vi "CRYGet Changed Ana Curve Name.vi"(0 "Old Name":string[](array[string]), 1 "Signal Tyep":string, 3 "Use Channel Name?":bool caption="Use Channel Name", 5 "Current Name":string[](array[string]), 7 "Changed Name Table in":string[][](array[string]), 9 "New Custom Type( Channel case)":string[](array[string]), 11 "Change State":bool, 12 "Load?":bool, 14 "Change Use Channel":bool) -> (10 "Changed Name Table  out":string[][](array[string]))   [LabVIEW 2013]
panel:
  out "Array":string[][](array[string])
  out "Changed Curve in":string[][](array[string])
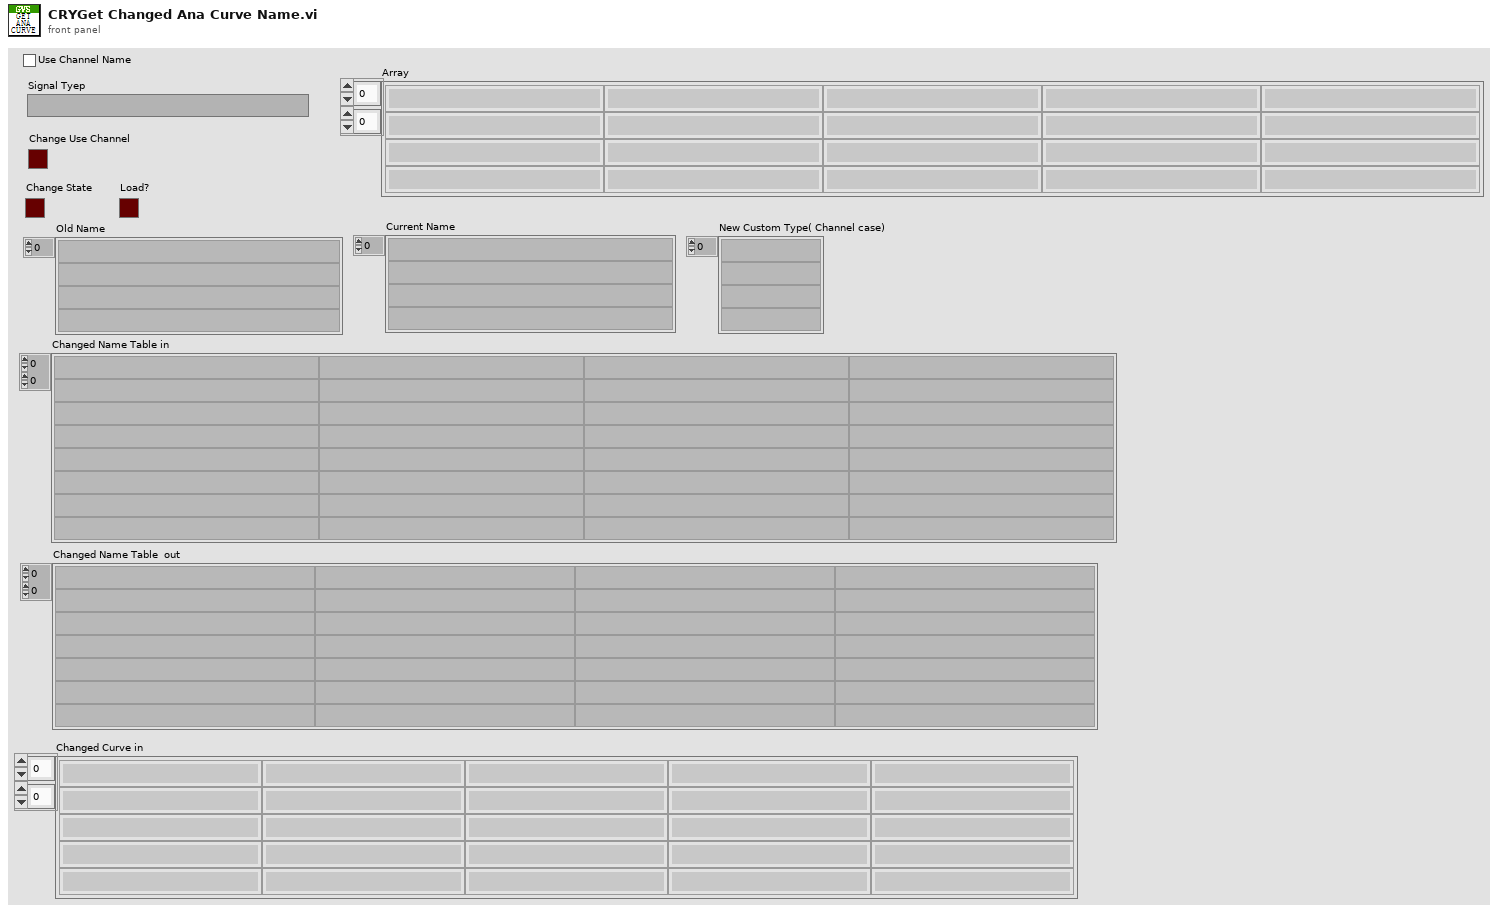
[diagram p1: front panel]
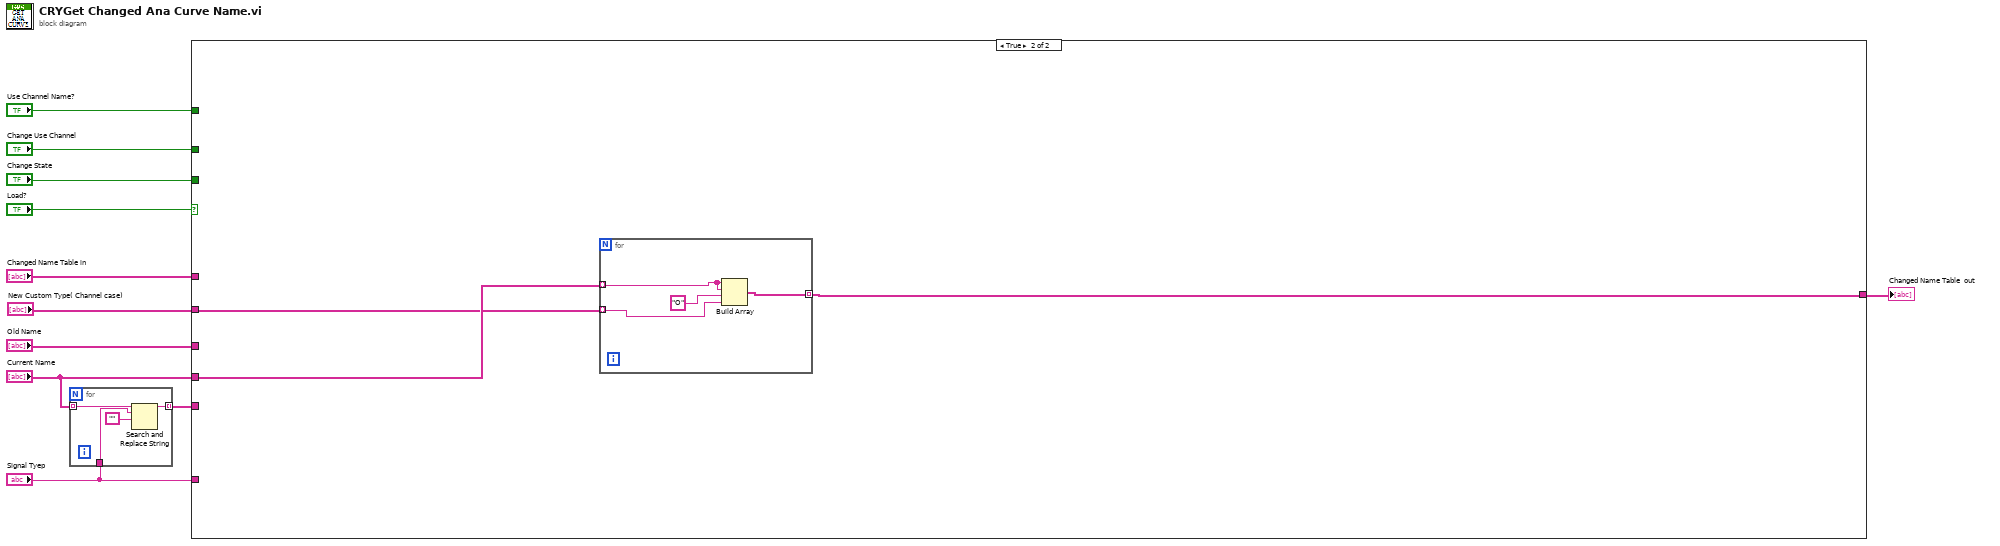
[diagram p0: block diagram]
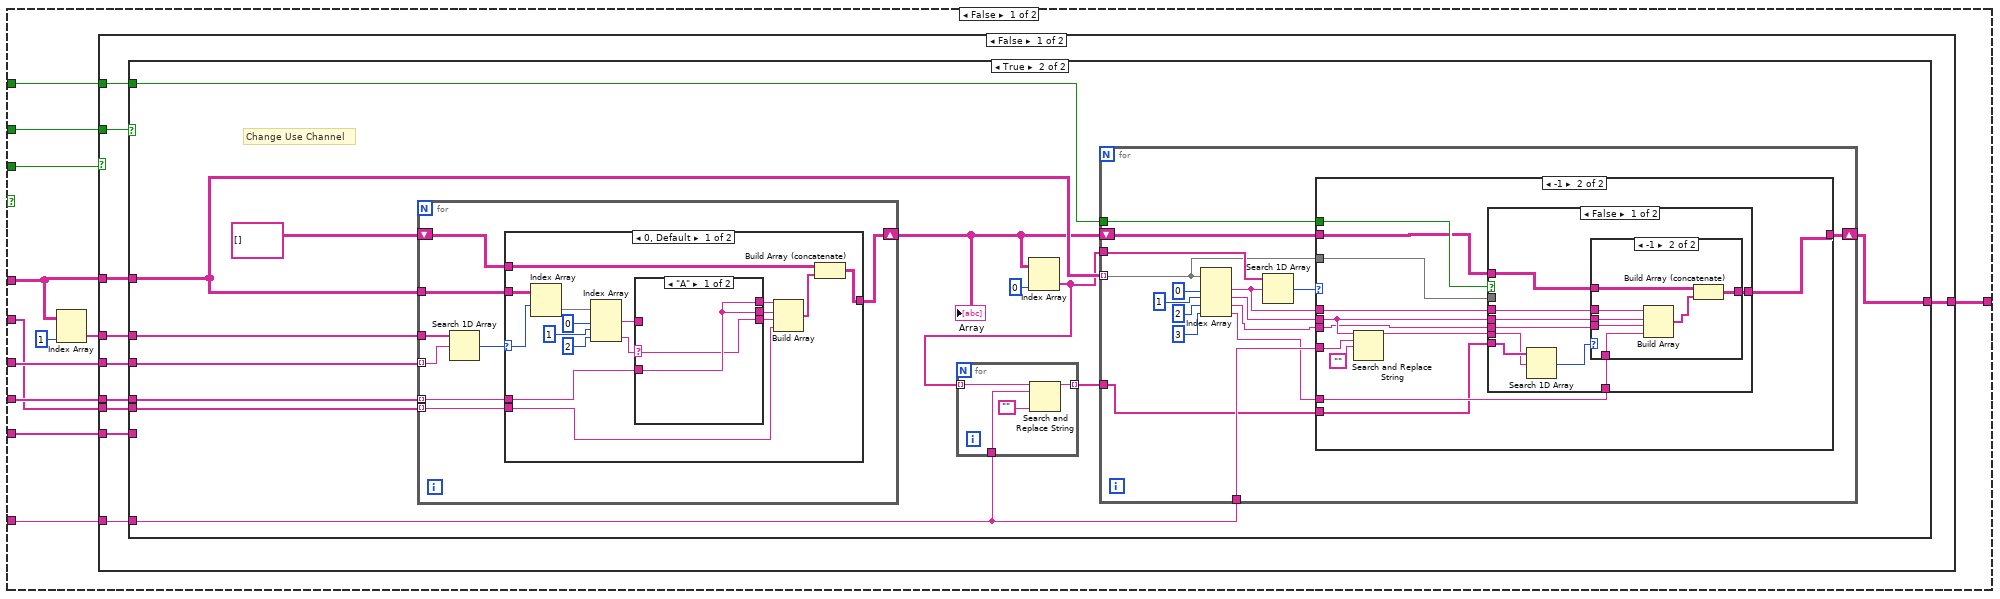
[diagram p2: hidden frame]
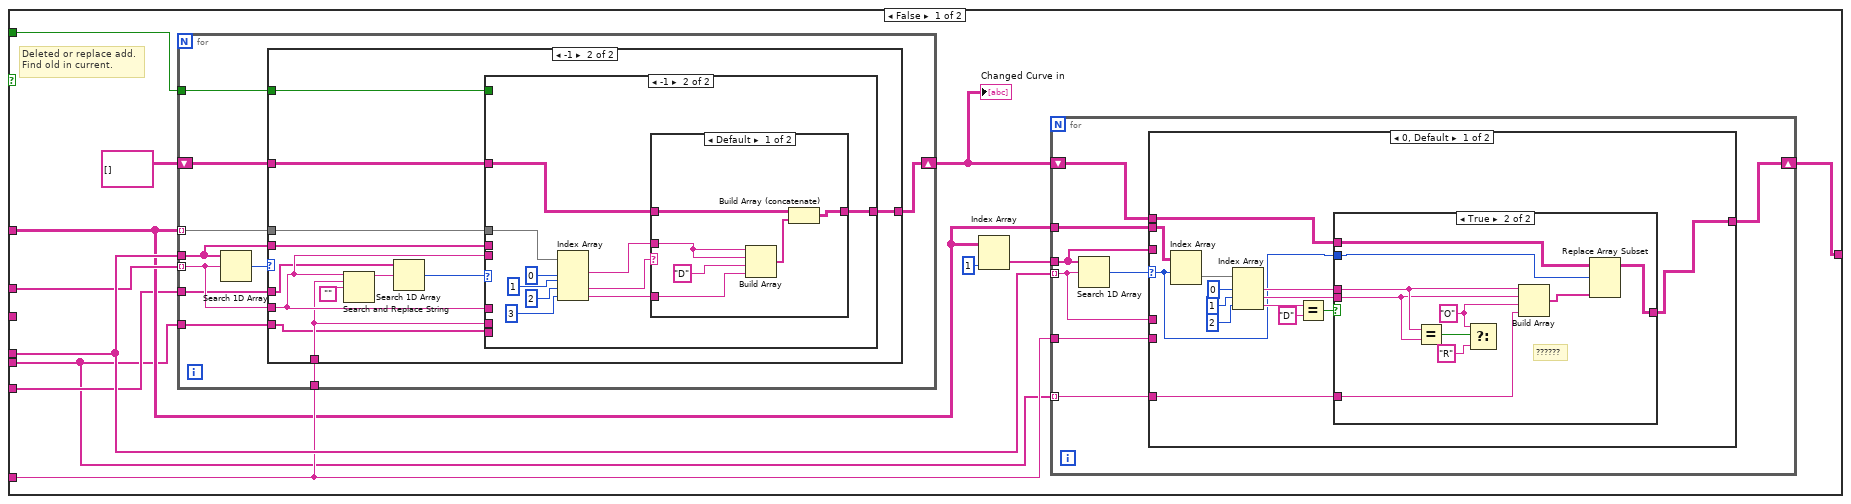
[diagram p3: hidden frame]
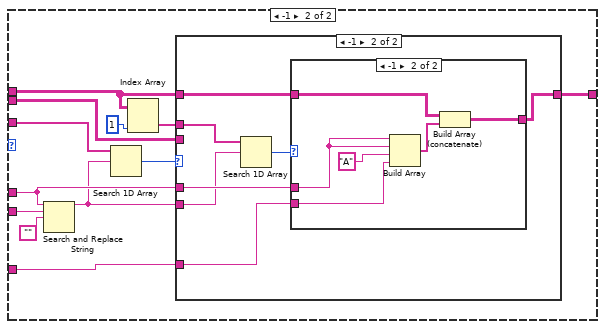
[diagram p5: hidden frame]
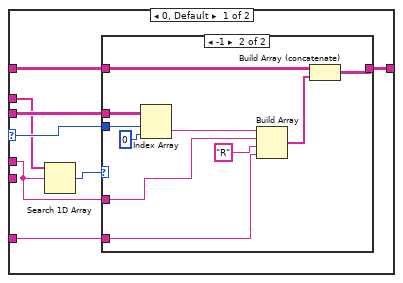
[diagram p6: hidden frame]
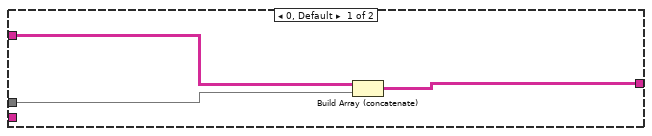
[diagram p9: hidden frame]
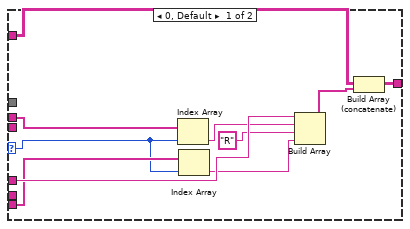
[diagram p10: hidden frame]
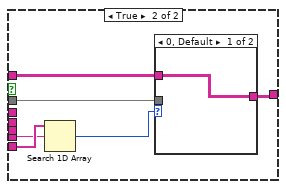
[diagram p14: hidden frame]
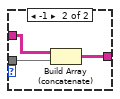
[diagram p15: hidden frame]
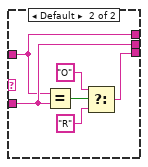
[diagram p16: hidden frame]
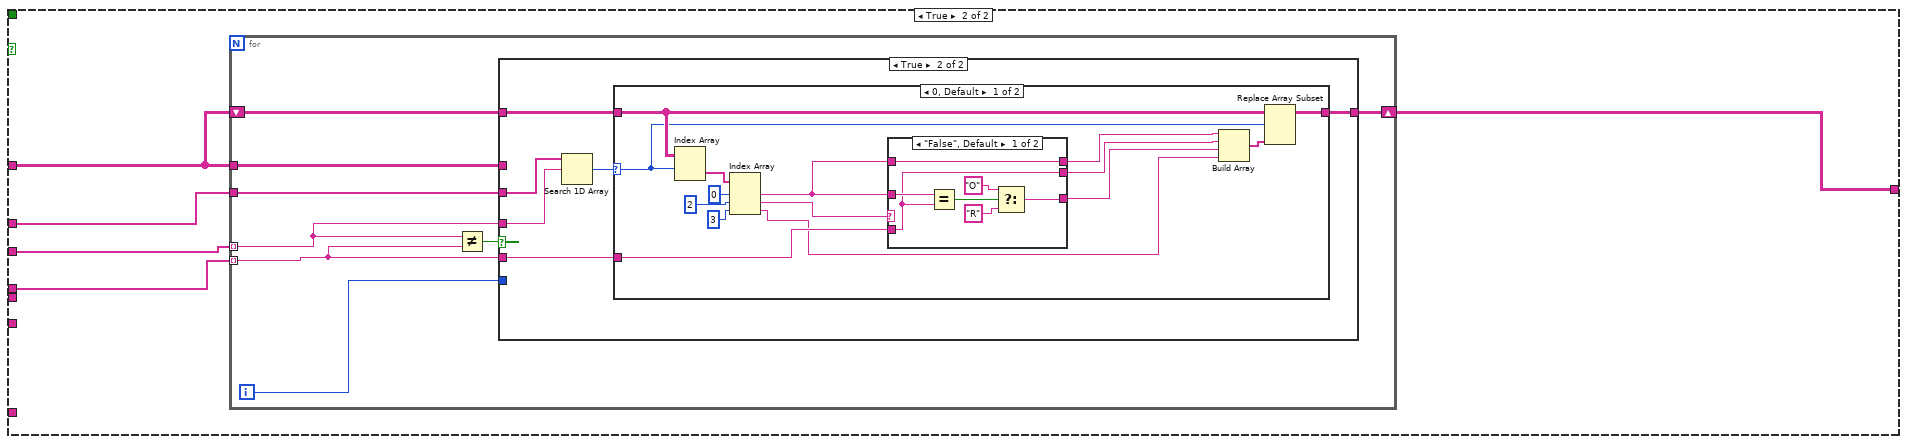
[diagram p18: hidden frame]
diagram:
  n1 = for {
    tunnel: "Current Name" -> [w14] mode=indexing
    tunnel: "Signal Tyep" -> [w13]
    tunnel: [w12] -> w2 mode=indexing
    n2 = Search and Replace String(input string=w14, search string=w13, replace string="" ("replace string (\"\")")) -> (result string=w12:string)  [unwired: 5 in, 3 out]
  }
  n3 = case shown="True" "Load?" {
    tunnel: [w27 w332] -> w11
    tunnel: "Changed Name Table in" -> [w25 _]
    tunnel: "Current Name" -> [w24 w333]
    tunnel: "Change State" -> [w23 _]
    tunnel: "Old Name" -> [w21 _]
    tunnel: "Change Use Channel" -> [w20 _]
    tunnel: "Signal Tyep" -> [w19 _]
    tunnel: "Use Channel Name?" -> [w18 _]
    tunnel: w2 -> [w17 _]
    tunnel: "New Custom Type( Channel case)" -> [w16 w331]
    frame False {
      n4 = Index Array(array=w25, index (col)=1 ("disabled index (col)")) -> (element=w22:string[])  [unwired: 1 in]
      n5 = case shown="False" w23 {
        tunnel: [w34 w286] -> w27
        tunnel: w22 -> [w36 w289]
        tunnel: w25 -> [w35 w287]
        tunnel: w24 -> [w37 w290]
        tunnel: w21 -> [w32 w288]
        tunnel: w20 -> [w33 _]
        tunnel: w19 -> [w31 _]
        tunnel: w18 -> [w30 _]
        tunnel: w17 -> [w29 _]
        tunnel: w16 -> [w28 _]
        frame False {
          n6 = case shown="True" w33 {
            tunnel: w37 -> [w48 w191]
            tunnel: w36 -> [w44 w189]
            tunnel: w35 -> [w40 w188]
            tunnel: [w47 w185] -> w34
            tunnel: w32 -> [_ w192]
            tunnel: w31 -> [w46 w182]
            tunnel: w30 -> [w45 w184]
            tunnel: w29 -> [w39 _]
            tunnel: w28 -> [w38 w183]
            frame False {
              # "Deleted or replace add.\nFind old in current."
              n7 = for {
                tunnel: w48 -> [w131]
                tunnel: w44 -> [w130] mode=indexing
                shift-right: [w136] -> w42
                shift-left: string[][] [] ("Changed Curve in") -> [w135]
                tunnel: w40 -> [w134] mode=indexing
                tunnel: w46 -> [w133]
                tunnel: w45 -> [w132]
                tunnel: w39 -> [w129]
                tunnel: w38 -> [w128]
                n8 = Search 1D Array(1D array=w131, element=w130) -> (index of element=w137:i32)  [unwired: 1 in]
                n9 = case shown="-1" w137 {
                  tunnel: [w139 w151] -> w136
                  tunnel: w135 -> [w140 w152]
                  tunnel: w134 -> [w138 w147]
                  tunnel: w133 -> [_ w143]
                  tunnel: w130 -> [_ w144]
                  tunnel: w132 -> [_ w145]
                  tunnel: w131 -> [_ w146]
                  tunnel: w129 -> [_ w142]
                  tunnel: w128 -> [_ w141]
                  frame 0, Default {
                    n10 = Build Array (concatenate)(w140, w138) -> (w139:string[][])
                  }
                  frame -1 {
                    n11 = Search and Replace String(input string=w144, search string=w143, replace string="" ("replace string (\"\")")) -> (result string=w149:string)  [unwired: 5 in, 3 out]
                    n12 = Search 1D Array(1D array=w142, element=w149) -> (index of element=w148:i32)  [unwired: 1 in]
                    n13 = case shown="-1" w148 {
                      selector: w148 -> [w154 _]
                      tunnel: w152 -> [w162 w172]
                      tunnel: [w161 w171] -> w151
                      tunnel: w147 -> [_ w167]
                      tunnel: w144 -> [w160 _]
                      tunnel: w145 -> [_ _]
                      tunnel: w143 -> [_ _]
                      tunnel: w146 -> [w159 _]
                      tunnel: w144 -> [_ _]
                      tunnel: w141 -> [w155 _]
                      frame 0, Default {
                        n14 = Index Array(array=w159, index=w154) -> (element=w156:string)
                        n15 = Index Array(array=w155, index=w154) -> (element=w153:string)
                        n16 = Build Array(w160, w156, "R" ("element"), w153) -> (w158:string[])
                        n17 = Build Array (concatenate)(w162, w158) -> (w161:string[][])
                      }
                      frame -1 {
                        n18 = Index Array(array=w167, index #1=0 ("index"), index #2=1 ("index"), index #3=2 ("index"), index #4=3 ("index")) -> (element #1=w166:string, element #3=w165:string, element #4=w163:string)  [unwired: 1 out]
                        n19 = case shown="Default" w165 {
                          tunnel: w172 -> [w178 w179]
                          tunnel: [w177 w179] -> w171
                          tunnel: w166 -> [w174 _]
                          tunnel: w163 -> [w173 _]
                          frame Default {
                            n20 = Build Array(w174, w174, "D" ("element"), w173) -> (w175:string[])
                            n21 = Build Array (concatenate)(w178, w175) -> (w177:string[][])
                          }
                          frame "A" {
                          }
                        }
                      }
                    }
                  }
                }
              }
              "Changed Curve in" <- w42
              n22 = Index Array(array=w40, index (col)=1 ("disabled index (col)")) -> (element=w41:string[])  [unwired: 1 in]
              n23 = for {
                tunnel: w48 -> [w53] mode=indexing
                shift-right: [w54] -> w47
                shift-left: w42 -> [w57]
                tunnel: w41 -> [w51]
                tunnel: w40 -> [w56]
                tunnel: w46 -> [w52]
                tunnel: w38 -> [w50] mode=indexing
                n24 = Search 1D Array(1D array=w51, element=w53) -> (index of element=w55:i32)  [unwired: 1 in]
                n25 = case shown="0, Default" w55 {
                  selector: w55 -> [w60 _]
                  tunnel: w57 -> [w61 w87]
                  tunnel: w56 -> [w71 w91]
                  tunnel: [w59 w86] -> w54
                  tunnel: w53 -> [_ w89]
                  tunnel: w52 -> [_ w93]
                  tunnel: w51 -> [_ w90]
                  tunnel: w50 -> [w58 w83]
                  frame 0, Default {
                    n26 = Index Array(array=w71, index (row)=w60) -> (element=w70:string[])  [unwired: 1 in]
                    n27 = Index Array(array=w70, index #1=0 ("index"), index #2=1 ("index"), index #3=2 ("index")) -> (element #1=w63:string, element #2=w62:string, element #3=w66:string)
                    n28 = Equal?(x=w66, y="D") -> (x = y?=w64:bool)
                    n29 = case shown="True" w64 {
                      tunnel: [w72 w77] -> w59
                      tunnel: w63 -> [_ w82]
                      tunnel: w62 -> [_ w81]
                      tunnel: w61 -> [w72 w79]
                      tunnel: w60 -> [_ w78]
                      tunnel: w58 -> [_ w73]
                      frame False {
                      }
                      frame True {
                        w74 = "O" ("element")
                        # "??????"
                        n30 = Equal?(x=w82, y=w81) -> (x = y?=w76:bool)
                        n31 = Select(t=w74, s=w76, f="R" ("element")) -> ()  [unwired: 1 out]
                        n32 = Build Array(w82, w81, w74, w73) -> (w80:string[])
                        n33 = Replace Array Subset(array=w79, new element=w80, index (row)=w78) -> (w77:string[][])  [unwired: 1 in]
                      }
                    }
                  }
                  frame -1 {
                    n34 = Search and Replace String(input string=w89, search string=w93, replace string="" ("replace string (\"\")")) -> (result string=w84:string)  [unwired: 5 in, 3 out]
                    n35 = Search 1D Array(1D array=w90, element=w84) -> (index of element=w92:i32)  [unwired: 1 in]
                    n36 = Index Array(array=w87, index (col)=1 ("disabled index (col)")) -> (element=w85:string[])  [unwired: 1 in]
                    n37 = case shown="-1" w92 {
                      selector: w92 -> [w101 _]
                      tunnel: w89 -> [w96 w120]
                      tunnel: w91 -> [w102 _]
                      tunnel: w87 -> [w98 w118]
                      tunnel: [w97 w119] -> w86
                      tunnel: w85 -> [w99 w117]
                      tunnel: w84 -> [_ w116]
                      tunnel: w83 -> [w95 w114]
                      frame 0, Default {
                        n38 = Search 1D Array(1D array=w99, element=w96) -> (index of element=w100:i32)  [unwired: 1 in]
                        n39 = case shown="-1" w100 {
                          tunnel: w102 -> [_ w113]
                          tunnel: w101 -> [_ w112]
                          tunnel: w98 -> [w103 w107]
                          tunnel: [w103 w105] -> w97
                          tunnel: w96 -> [_ w109]
                          tunnel: w95 -> [_ w104]
                          frame 0, Default {
                          }
                          frame -1 {
                            n40 = Index Array(array=w113, index (row)=w112, index (col)=0 ("disabled index (col)")) -> (element=w110:string)
                            n41 = Build Array(w110, w109, "R" ("element"), w104) -> (w106:string[])
                            n42 = Build Array (concatenate)(w107, w106) -> (w105:string[][])
                          }
                        }
                      }
                      frame -1 {
                        n43 = Search 1D Array(1D array=w117, element=w116) -> (index of element=w115:i32)  [unwired: 1 in]
                        n44 = case shown="-1" w115 {
                          tunnel: w120 -> [_ w127]
                          tunnel: [w121 w124] -> w119
                          tunnel: w118 -> [w121 w123]
                          tunnel: w114 -> [_ w122]
                          frame 0, Default {
                          }
                          frame -1 {
                            n45 = Build Array(w127, w127, "A" ("element"), w122) -> (w125:string[])
                            n46 = Build Array (concatenate)(w123, w125) -> (w124:string[][])
                          }
                        }
                      }
                    }
                  }
                }
              }
            }
            frame True {
              # "Change Use Channel"
              n47 = for {
                tunnel: w191 -> [w254] mode=indexing
                shift-right: [w256] -> w187
                shift-left: string[][] [] -> [w260]
                tunnel: w192 -> [w258] mode=indexing
                tunnel: w189 -> [w259]
                tunnel: w188 -> [w255]
                tunnel: w183 -> [w253] mode=indexing
                n48 = Search 1D Array(1D array=w259, element=w258) -> (index of element=w257:i32)  [unwired: 1 in]
                n49 = case shown="0, Default" w257 {
                  selector: w257 -> [w273 _]
                  tunnel: w260 -> [w276 w285]
                  tunnel: [w275 w285] -> w256
                  tunnel: w255 -> [w274 _]
                  tunnel: w254 -> [w268 _]
                  tunnel: w253 -> [w261 _]
                  frame 0, Default {
                    n50 = Index Array(array=w274, index (row)=w273) -> (element=w272:string[])  [unwired: 1 in]
                    n51 = Index Array(array=w272, index #1=0 ("index"), index #2=1 ("index"), index #3=2 ("index")) -> (element #1=w265:string, element #3=w262:string)  [unwired: 1 out]
                    n52 = case shown="\"A\"" w262 {
                      selector: w262 -> [w277 _]
                      tunnel: w265 -> [_ w279]
                      tunnel: w268 -> [w278 w280]
                      tunnel: [w277 w281] -> w267
                      tunnel: [w278 w279] -> w263
                      tunnel: [w278 w280] -> w264
                      frame "A" {
                      }
                      frame Default {
                        n53 = Equal?(x=w279, y=w280) -> (x = y?=w284:bool)
                        n54 = Select(t="O" ("Custom Curve Names"), s=w284, f="R" ("Custom Curve Names")) -> (s? t:f=w281:string)
                      }
                    }
                    n55 = Build Array(w263, w264, w267, w261) -> (w266:string[])
                    n56 = Build Array (concatenate)(w276, w266) -> (w275:string[][])
                  }
                  frame -1 {
                  }
                }
              }
              "Array" <- w187
              n57 = Index Array(array=w187, index (col)=0 ("disabled index (col)")) -> (element=w180:string[])  [unwired: 1 in]
              n58 = for {
                tunnel: w180 -> [w195] mode=indexing
                tunnel: w182 -> [w194]
                tunnel: [w193] -> w181 mode=indexing
                n59 = Search and Replace String(input string=w195, search string=w194, replace string="" ("replace string (\"\")")) -> (result string=w193:string)  [unwired: 5 in, 3 out]
              }
              n60 = for {
                shift-right: [w207] -> w185
                shift-left: w187 -> [w206]
                tunnel: w188 -> [w205] mode=indexing
                tunnel: w180 -> [w209]
                tunnel: w182 -> [w204]
                tunnel: w184 -> [w203]
                tunnel: w181 -> [w198]
                n61 = Index Array(array=w205, index #1=0 ("index"), index #2=1 ("index"), index #3=2 ("index"), index #4=3 ("index")) -> (element #1=w202:string, element #2=w201:string, element #3=w197:string, element #4=w199:string)
                n62 = Search 1D Array(1D array=w209, element=w202) -> (index of element=w208:i32)  [unwired: 1 in]
                n63 = case shown="-1" w208 {
                  tunnel: [w213 w216] -> w207
                  tunnel: w206 -> [w213 w215]
                  tunnel: w205 -> [_ w221]
                  tunnel: w204 -> [_ w224]
                  tunnel: w203 -> [_ w225]
                  tunnel: w202 -> [_ w220]
                  tunnel: w201 -> [_ w217]
                  tunnel: w199 -> [_ w219]
                  tunnel: w198 -> [_ w218]
                  tunnel: w197 -> [_ w214]
                  frame 0, Default {
                  }
                  frame -1 {
                    n64 = Search and Replace String(input string=w217, search string=w224, replace string="" ("replace string (\"\")")) -> (result string=w222:string)  [unwired: 5 in, 3 out]
                    n65 = case shown="False" w225 {
                      tunnel: w222 -> [w228 w247]
                      tunnel: w221 -> [_ w245]
                      tunnel: w220 -> [w234 _]
                      tunnel: w217 -> [w233 _]
                      tunnel: w219 -> [w232 _]
                      tunnel: w218 -> [w229 w248]
                      tunnel: w215 -> [w231 w244]
                      tunnel: [w230 w243] -> w216
                      tunnel: w214 -> [w226 _]
                      frame False {
                        n66 = Search 1D Array(1D array=w229, element=w228) -> (index of element=w227:i32)  [unwired: 1 in]
                        n67 = case shown="-1" w227 {
                          tunnel: w234 -> [_ w242]
                          tunnel: w233 -> [_ w241]
                          tunnel: w226 -> [_ w240]
                          tunnel: w232 -> [_ w239]
                          tunnel: w231 -> [w235 w238]
                          tunnel: [w235 w236] -> w230
                          frame 0, Default {
                          }
                          frame -1 {
                            n68 = Build Array(w242, w241, w240, w239) -> (w237:string[])
                            n69 = Build Array (concatenate)(w238, w237) -> (w236:string[][])
                          }
                        }
                      }
                      frame True {
                        n70 = Search 1D Array(1D array=w248, element=w247) -> (index of element=w246:i32)  [unwired: 1 in]
                        n71 = case shown="0, Default" w246 {
                          tunnel: w245 -> [_ w252]
                          tunnel: w244 -> [w249 w251]
                          tunnel: [w249 w250] -> w243
                          frame 0, Default {
                          }
                          frame -1 {
                            n72 = Build Array (concatenate)(w251, w252) -> (w250:string[][])
                          }
                        }
                      }
                    }
                  }
                }
              }
            }
          }
        }
        frame True {
          n73 = for {
            tunnel: w288 -> [w292] mode=indexing
            tunnel: w290 -> [w291] mode=indexing
            tunnel: w289 -> [w295]
            tunnel: w287 -> [w294]
            shift-right: [w296] -> w286
            shift-left: w287 -> [w297]
            i -> [w293]
            n74 = Not Equal?(x=w292, y=w291) -> (x != y?=w298:bool)
            n75 = case shown="True" w298 {
              tunnel: w292 -> [_ w301]
              tunnel: w291 -> [_ w303]
              tunnel: w297 -> [w299 w305]
              tunnel: [w299 w304] -> w296
              tunnel: w295 -> [_ w302]
              tunnel: w294 -> [_ _]
              tunnel: w293 -> [_ _]
              frame False {
              }
              frame True {
                n76 = Search 1D Array(1D array=w302, element=w301) -> (index of element=w300:i32)  [unwired: 1 in]
                n77 = case shown="0, Default" w300 {
                  selector: w300 -> [w314 _]
                  tunnel: w305 -> [w315 w330]
                  tunnel: [w316 w330] -> w304
                  tunnel: w303 -> [w319 _]
                  frame 0, Default {
                    n78 = Index Array(array=w315, index (row)=w314) -> (element=w313:string[])  [unwired: 1 in]
                    n79 = Index Array(array=w313, index #1=0 ("index"), index #2=2 ("index"), index #3=3 ("index")) -> (element #1=w310:string, element #2=w311:string, element #3=w306:string)
                    n80 = case shown="\"False\", Default" w311 {
                      selector: w311 -> [_ w328]
                      tunnel: w310 -> [w326 _]
                      tunnel: w319 -> [w321 w329]
                      tunnel: [w323 w328] -> w318
                      tunnel: w310 -> [w322 _]
                      tunnel: [w322 w329] -> w309
                      tunnel: [w321 w329] -> w308
                      frame "False", Default {
                        n81 = Equal?(x=w326, y=w321) -> (x = y?=w327:bool)
                        n82 = Select(t="O" ("Custom Curve Names"), s=w327, f="R" ("Custom Curve Names")) -> (s? t:f=w323:string)
                      }
                      frame "A" {
                      }
                    }
                    n83 = Build Array(w309, w308, w318, w306) -> (w317:string[])
                    n84 = Replace Array Subset(array=w315, new element=w317, index (row)=w314) -> (w316:string[][])  [unwired: 1 in]
                  }
                  frame -1 {
                  }
                }
              }
            }
          }
        }
      }
    }
    frame True {
      n85 = for {
        tunnel: [w337] -> w332 mode=indexing
        tunnel: w333 -> [w336] mode=indexing
        tunnel: w331 -> [w334] mode=indexing
        n86 = Build Array(w336, w336, "O" ("Custom Curve Names"), w334) -> (w337:string[])
      }
    }
  }
  "Changed Name Table  out" <- w11
